vi "Pendel.vi"() -> ()   [LabVIEW 2014]
uses:
  Reglertyp.ctl
  <vilib>/Platform/TimedLoop/XDataNode/timing_clust.ctl
  <vilib>/Platform/TimedLoop/XDataNode/nitl_modes.ctl
  <vilib>/Platform/TimedLoop/XDataNode/wakeup.ctl
  <vilib>/Simulation/Scripting/Companion Diagram/SimConfigNode/SimParams.ctl
  <vilib>/Simulation/Scripting/Companion Diagram/SimConfigNode/_simSolvers.ctl
  <vilib>/Simulation/Implementation/Shared/SIMSCR Execution Mode.ctl
  <vilib>/Simulation/Param Hierarchy/Typedefs/SIMPH Param Control Actions.ctl
  <vilib>/Statechart/Common/IntGuid.ctl
  <vilib>/Statechart/Common/DbgID.ctl
  <vilib>/Analysis/baseanly.llb/Real A x B.vi
  <vilib>/Simulation/Implementation/Shared/NILVSim_ParamChanged.vi
  <vilib>/Simulation/Implementation/Shared/NILVSIM_BeginStep.vi
  <vilib>/Simulation/Implementation/Shared/NILVSim_Manager.vi
  <vilib>/Utility/error.llb/Clear Errors.vi
  <vilib>/Simulation/Implementation/Shared/NILVSim_FinalizeModel.vi
  Pendel.lvsc/CompanionDiagram.vi
  Pendel.lvsc/CompanionDiagram.vi/21/SC Main.vi
  <vilib>/Simulation/Implementation/Shared/SIM Unbundle Sim Info.vi
  <vilib>/Simulation/Implementation/Shared/NILVSim_Initialize.vi
  <vilib>/Simulation/Utility/Implementation/NILVSim Get Time and IsAcceptedStep.vi
  <vilib>/Simulation/Implementation/Shared/SIMSH Read Queue.vi
  <vilib>/Simulation/Implementation/Shared/NILVSim_GetModelError.vi
  <vilib>/Simulation/Implementation/Shared/SIM Bundle Sim Info.vi
  Pendel.lvsc/Trigger.ctl
  <vilib>/Statechart/Infrastructure/RTStatechart/RunTime SCN.xnode
  Pendel.lvsc/Inputs.ctl
  Pendel.lvsc/Outputs.ctl
  Pendel.lvsc
  <vilib>/Platform/TimedLoop/XDataNode/XDataNode.xnode
  <vilib>/Simulation/Implementation/XNodeFramework/SimXNode/SimX.xnode
  <vilib>/Simulation/Scripting/Companion Diagram/SimConfigNode/SimDog.xnode
  <vilib>/Platform/TimedLoop/XDataNode/XDNodeRunTimeDep.lvlib
  <vilib>/Analysis/NI_AALBase.lvlib
  <vilib>/ptbypt/NI_PtbyPt.lvlib
  <vilib>/Statechart/Common/NI_SC_LVSCCommonFiles.lvlib
  <vilib>/Simulation/Implementation/Shared/NI_SIM_Implementation.lvlib
panel:
  out "Winkel 1":dbl
  out "Geschwindigkeit":dbl
  out "Position":dbl
  out "Winkel2":dbl
  out "Winkelgeschwindigkeit2":dbl
  out "Winkelgeschwindigkeit1":dbl
  out "Kraft berechnet":cluster{"Kraft (N)":dbl, dbl}(graph)
  out "Schleifendauer":i64(graph)
  in  "Registerkarte":enum32{"Pendel", "S706", "Wegzähler"}(tab)
  in  "Reglertyp":T1
  in  "Positionieren":bool
  out "Kraft (N)":dbl(graph)
  out "Winkel (Grad)":cluster{"Double":dbl, "Double":dbl}(graph)
  in  "Schließen":bool
  in  "Regler anhalten":bool
  in  "Regler starten":bool
  in  "Ruhelage":bool=TRUE
  in  "Pendelaufbau":T2(ring)
  out "Aktueller Zustand":string
  in  "Referenzieren":bool
  in  "Sollposition (mm)":dbl(slide) scale=-500.0..500.0
  out "Position (mm)":T3(graph)
  out "S706 Status (SDO 6041)":T4
  in  "S706 parametrieren":bool
  out "S706":string
  out "Wegzähler (m)":dbl
  out "Wegzähler (m)":dbl(knob)=6.6072914947233965 scale=5000.0..5000000.0
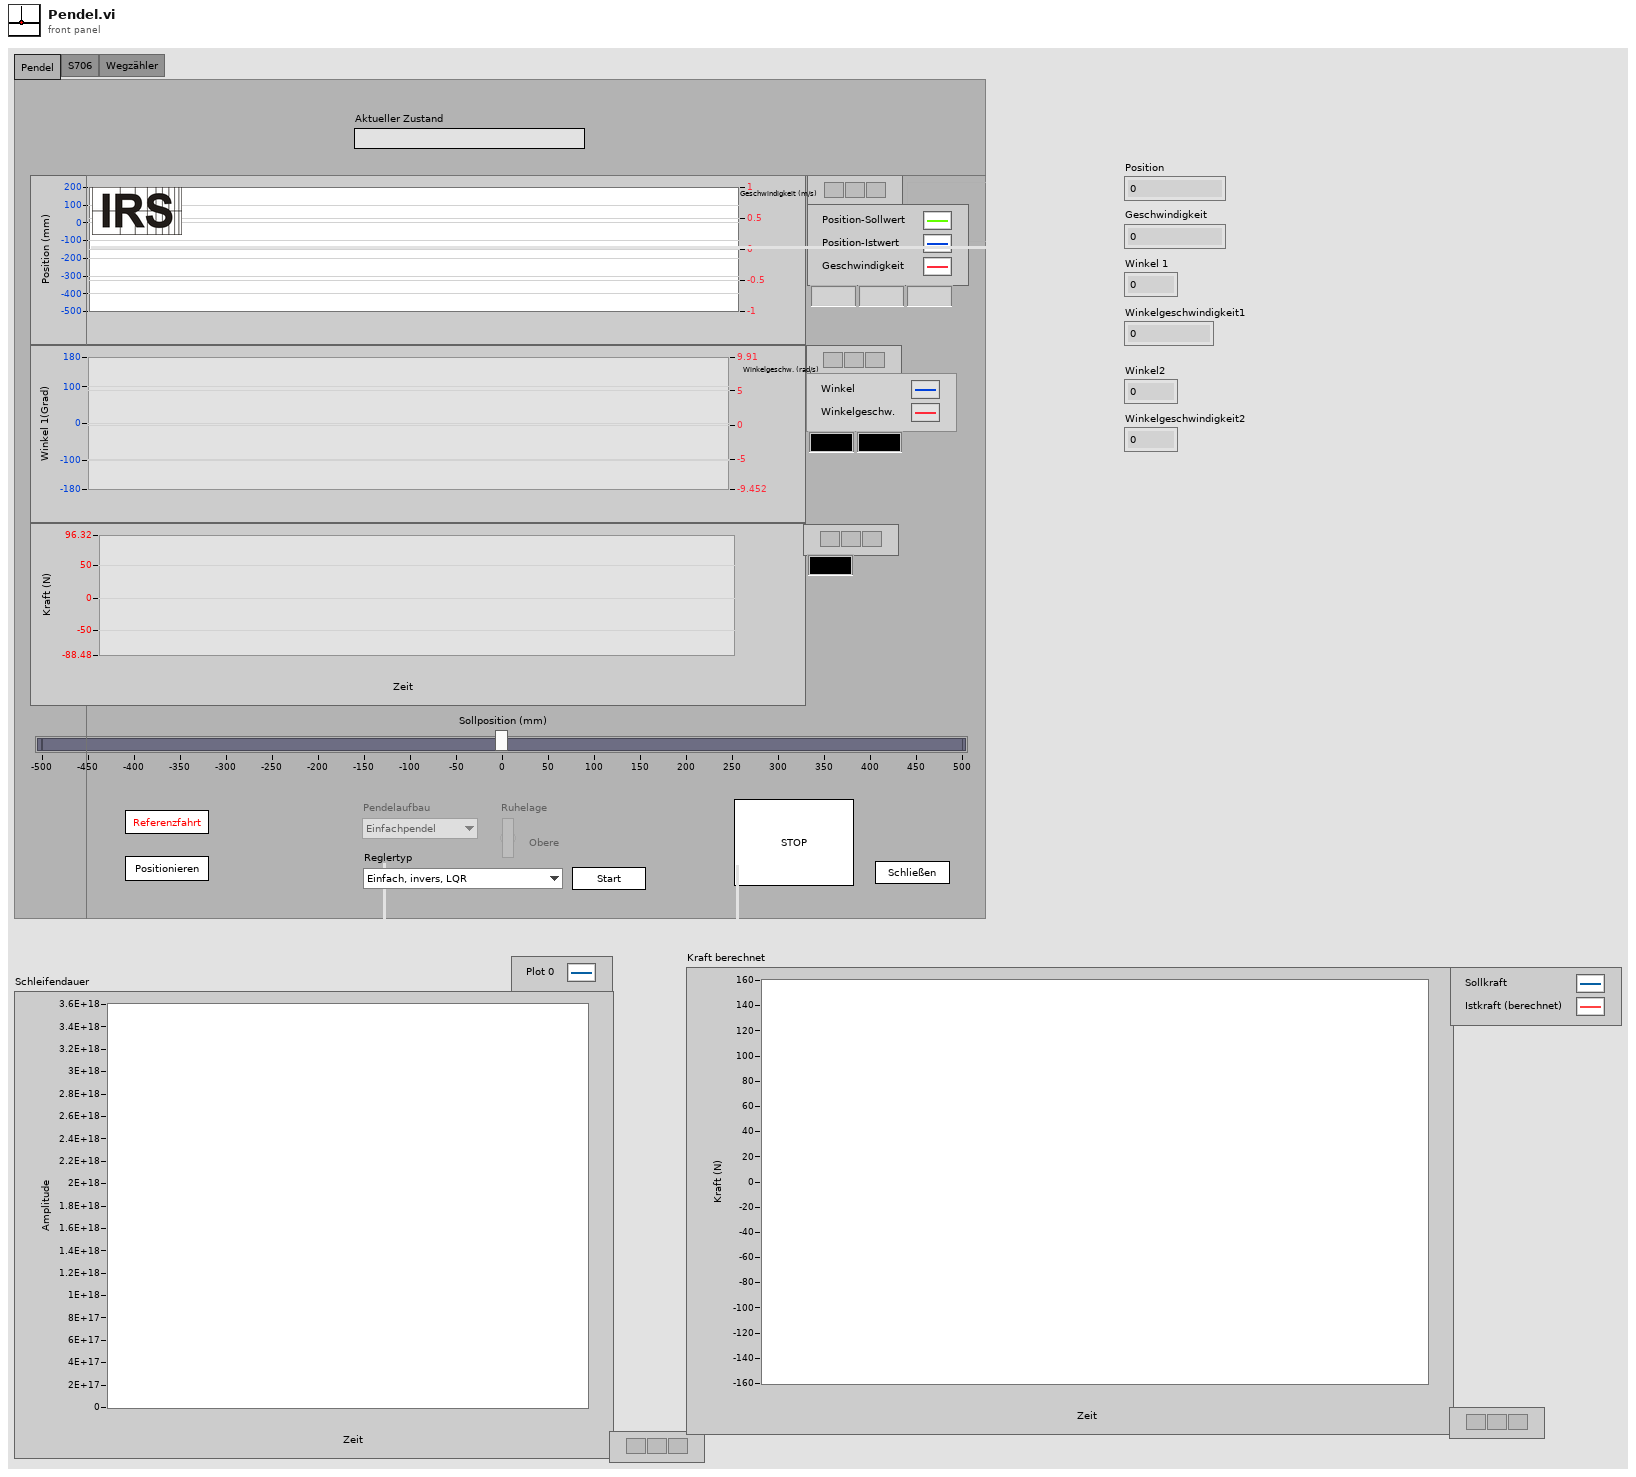
[diagram p1: front panel]
types:
  T1 = typedef "Reglertyp.ctl" = enum16{"Einfach, invers, LQR", "Einfach, invers, Kaskade", "Doppelt, invers, LQR"}
  T2 = enum16{"Einfachpendel", "Doppelpendel", "Dreifachpendel"}
  T3 = cluster{"Sollposition (mm)":dbl, dbl, "Double":dbl}
  T4 = cluster{"0 ready to switch on":bool, "1 switched on":bool, "2 operation enable":bool, "3 fault":bool, "4 voltage enabled":bool, "5 quick stop":bool, "6 switch on disable":bool, "7 warning":bool, "8 ":bool, "9 remote (kann kommunizieren)":bool, "10 target_reached":bool, "11 internal_limit_active":bool, "12 Referenzfahrt durchgeführt":bool, "13 Referenzfahrtfehler":bool}
  T5 = cluster{"Pendelaufbau":enum16{"Einfachpendel", "Doppelpendel", "Dreifachpendel"}, "Winkel1":refnum<k21>, "Winkel2":refnum<k21>, "Winkel3":refnum<k21>}
  T6 = cluster{"node-ID":u8, "RPDO1 controlword":refnum<k20>, "TPDO1 status":refnum<k20>, "RPDO2 I-Sollwert":refnum<k20>, "TPDO2 Ist-Werte":refnum<k20>, "SYNC object":refnum<k20>}
  T7 = typedef "XDNodeRunTimeDep.lvlib/timing_clust.ctl" = cluster{"Expected End [f-1]":u64, "Actual End [f-1]":u64, "Finished Late? [f-1]":bool, "Expected End [i-1]":u64, "Actual End [i-1]":u64, "Finished Late? [i-1]":bool, "Expected Start [i]":u64, "Actual Start [i]":u64, "Expected Start [f]":u64, "Actual Start [f]":u64, "Source Name":string, "Structure Name":string, "Period":i64, "Deadline":i64, "Offset":i64, "Start":i64, "Priority":i32, "Timeout":i32, "Mode":T8, "Wakeup Reason":T9, "Error":errorcluster, "Source Type":string, "Secondary Source Type":string, "Global End Time":u64, "Global Start Time":u64, "Frame Duration":u64, "Iteration Duration":u64, "Assigned CPU":i32, "I/O Scan Engine Mode":u32}
  T8 = typedef "XDNodeRunTimeDep.lvlib/nitl_modes.ctl" = enum32{"No Change", "Process missed periods, maintain original phase", "Discard missed periods, maintain original phase", "Process missed periods, ignore original phase", "Discard missed periods, ignore original phase"}
  T9 = typedef "XDNodeRunTimeDep.lvlib/wakeup.ctl" = enum32{"Normal", "Aborted", "Asynchronous wakeup", "Timing source error", "Timed loop error", "Timeout"}
  T10 = enum16{"Simulate to Completion", "Single Time-Step Simulation (Fixed Step Only)"}
  T11 = typedef "SIMSCR Execution Mode.ctl" = enum16{"Simulate to Completion", "Single Time-Step Simulation (Fixed Step Only)"}
  T12 = typedef "SIMPH Param Control Actions.ctl" = enum16{"get params", "set params"}
  T13 = cluster{"SIMSH Sim Time":dbl, "Saturation":cluster{"output":dbl}, "Derivative":cluster{"output":dbl}, "Integrator":cluster{"output":dbl}, "Transfer Function":cluster{"output y(t)":dbl}, "Summation 7":cluster{"Result":dbl}, "Gain 3":cluster{"output":dbl}, "Gain 2":cluster{"output":dbl}, "Summation 4":cluster{"Result":dbl}, "Summation 6":cluster{"Result":dbl}}
  T14 = typedef "SimParams.ctl" = cluster{"Initial Time (s)":dbl, "Final Time (s)":dbl, "Step Size (s)":dbl, "ODE Solver":T15, "Minimum Step Size (s)":dbl, "Maximum Step Size (s)":dbl, "Relative Tolerance":dbl, "Absolute Tolerance":dbl, "Software Timing":bool, "Initial Step Size (s)":dbl, "Automatic Fixed Step Size?":bool, "Automatic Discrete Step Size?":bool, "Discrete Step Size (s)":dbl, "Calculate using Time Step":bool, "Solver Wired?":bool, "Prev.Frm.Expected End":u64, "Prev.Frm.Actual End":u64, "Prev.Frm.Finished Late?":bool, "Prev.Iter.Expected End":u64, "Prev.Iter.Actual End":u64, "Prev.Iter.Finished Late?":bool, "Expected Iteration Start":u64, "Actual Iteration Start":u64, "Expected Frame Start":u64, "Actual Frame Start":u64, "Source Name":string, "Name":string, "Period":i64, "Deadline":i64, "Offset":i64, "Start":i64, "Priority":i32, "Timeout":i32, "Processor":i32, "Mode":enum32{"No Change", "Process missed periods, maintain original phase", "Discard missed periods, maintain original phase", "Process missed periods, ignore original phase", "Discard missed periods, ignore original phase"}, "Wakeup reason":enum32{"Normal", "Aborted", "Asynchronous wakeup", "Timing source error", "Timed loop error", "Timeout"}, "Error":errorcluster, "Source Type":string, "Secondary Source Type":string, "Global End Time":u64, "Global Start Time":u64, "Full Solver Reset":bool, "Execution Mode":T11, "Nan/Inf Check":bool, "Custom Solver Library":string, "Solver Is Variable":bool, "custom solver name":string, "Signal Collection Decimation":u32}
  T15 = typedef "_simSolvers.ctl" = enum16{"Runge-Kutta 1 (Euler)", "Runge-Kutta 2", "Runge-Kutta 3", "Runge-Kutta 4", "Runge-Kutta 23 (variable)", "Runge-Kutta 45 (variable)", "BDF (variable)", "Adams-Moulton (variable)", "Rosenbrock (variable)", "Discrete States Only", "SDIRK 4 (variable)", "Radau 5 (variable)", "Radau 9 (variable)", "Radau 13 (variable)", "Radau [Variable Order] (variable)", "Gear's Method (variable)", "Linearizer", "State Query", "Trim Eval", "Custom Solver"}
  T16 = cluster{"Winkel1":dbl, "Winkel2":dbl, "Winkel3":dbl}
  T17 = cluster{"Winkelgeschwindigkeit1":dbl, "Winkelgeschwindigkeit2":dbl, "Winkelgeschwindigkeit3":dbl}
  T18 = typedef "NI_Matrix.lvlib/RealMatrix.ctl" = dbl[][]
  T19 = typedef "NI_SC_LVSCCommonFiles.lvlib/IntGuid.ctl" = cluster{"Data1":u32, "Data2":u16, "Data3":u16, "Data4":u8, "Data5":u8, "Data6":u8, "Data11":u8, "Data9":u8, "Data10":u8, "Data8":u8, "Data7":u8}
  T20 = typedef "NI_SC_LVSCCommonFiles.lvlib/DbgID.ctl" = cluster{"VIRef":u32, "IntGUID":T19}
  T21 = enum16{"unbekannt", "Quick stop active", "Fault reaction active", "Fault", "Operation enabled", "Switched on", "Ready to switch on", "Switch on disabled", "Not Ready to switch on"}
  T22 = cluster{bool, bool, bool, bool, bool, bool, bool, bool, bool, bool, bool, bool, bool, bool}
  T23 = cluster{"Positionieren":bool, "Referenzieren":bool, "Regler darf starten":bool, "Regler anhalten":bool, "Schließen":bool, "S706 parametrieren":bool, "error out":errorcluster}
  T24 = typedef "Pendel.lvsc/Outputs.ctl" = cluster{"Zustand":string, "error out":errorcluster}
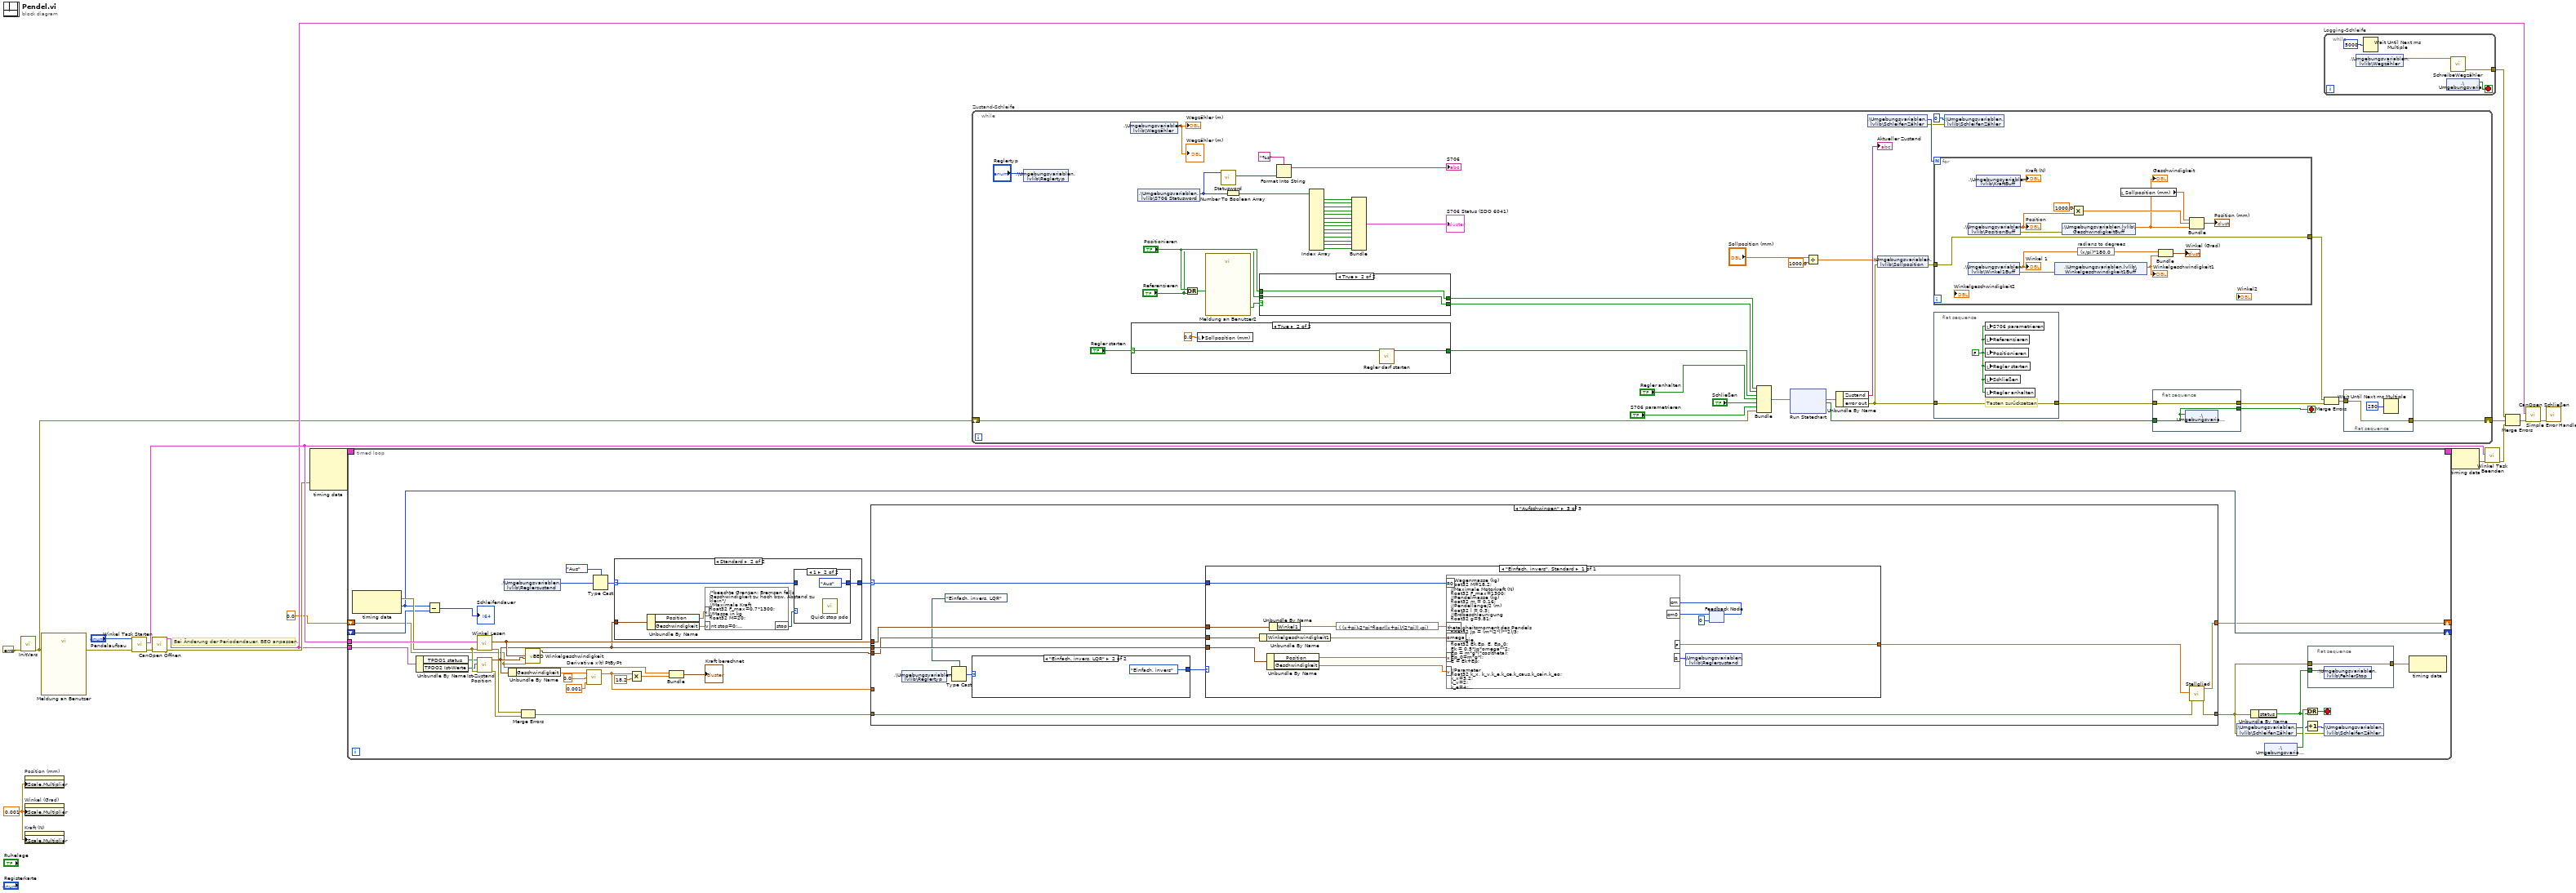
[diagram p0: block diagram]
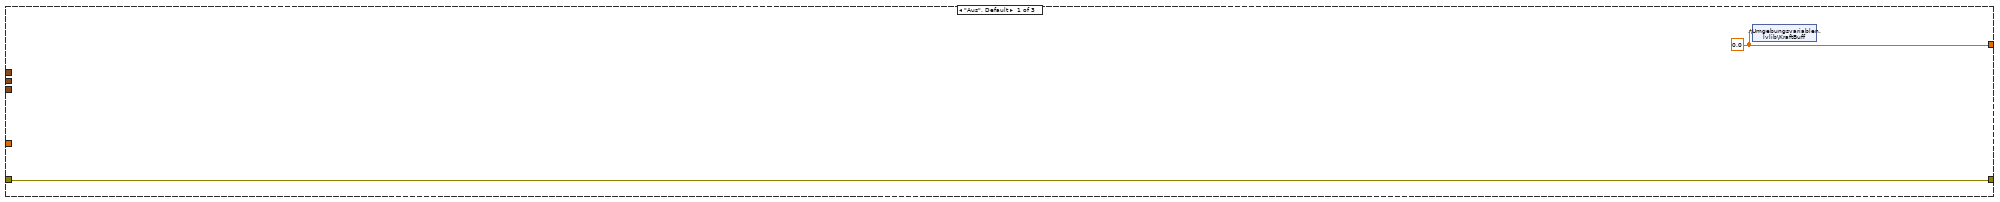
[diagram p4: hidden frame]
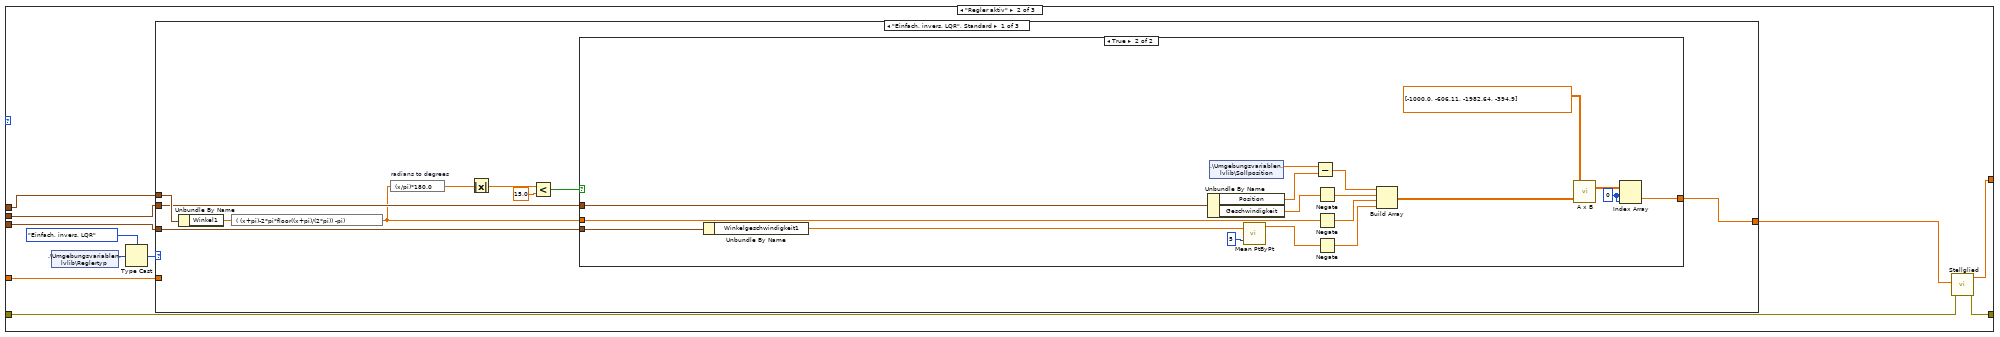
[diagram p5: hidden frame]
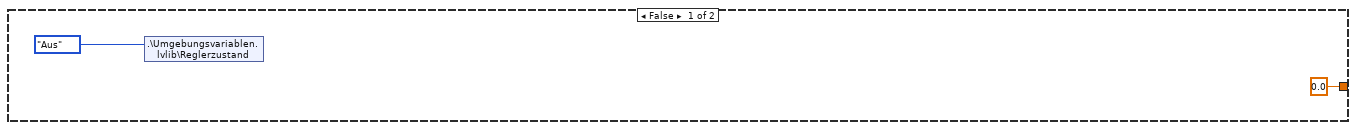
[diagram p6: hidden frame]
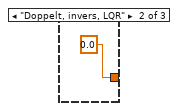
[diagram p7: hidden frame]
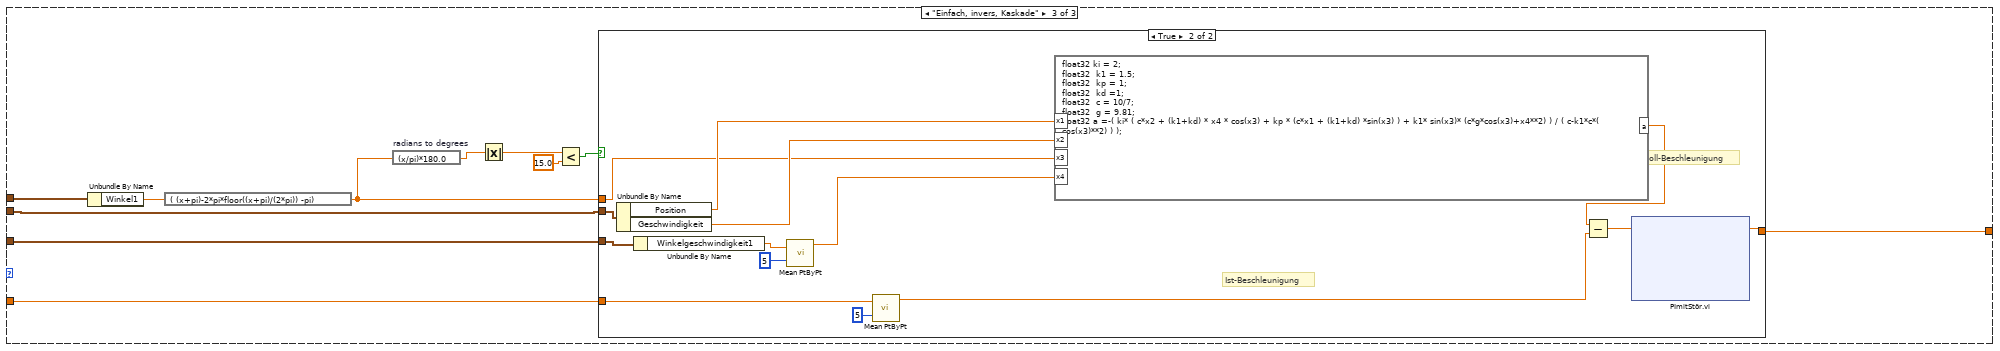
[diagram p8: hidden frame]
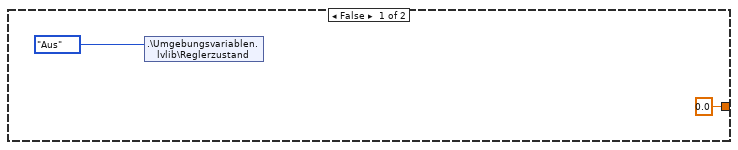
[diagram p9: hidden frame]
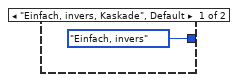
[diagram p10: hidden frame]
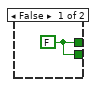
[diagram p11: hidden frame]
diagram:
  w5 = 0.001 ("X-Achse.Offset und Faktor:Faktor")
  # "Bei Änderung der Periodendauer, BEO anpassen."
  n1 = call "InitVars.vi"("error in (no error)"=errorcluster {"status"=FALSE, "code"=0, "source"=""} ("error IO")) -> ("error out"=w4:errorcluster)  [unwired: 10 in]
  n2 = property on="Position (mm)" class="SVDiagr (strikt)"("XScale.Multiplier"=w5) -> ()  [unwired: 2 in, 2 out]
  n3 = property on="Winkel (Grad)" class="SVDiagr (strikt)"("XScale.Multiplier"=w5) -> ()  [unwired: 2 in, 2 out]
  n4 = property on="Kraft (N)" class="SVDiagr (strikt)"("XScale.Multiplier"=w5) -> ()  [unwired: 2 in, 2 out]
  n5 = call "Meldung an Benutzer"("error in (no error)"=w4) -> ("error out"=w10:errorcluster)  [unwired: 9 in, 1 out]
  n6 = call "Winkel Task Starten.vi"("error IO"=w10, "Pendelaufbau in"="Pendelaufbau") -> ("error out"=w2:errorcluster, "Winkel Task"=w13:T5)  [unwired: 8 in]
  n7 = call "CanOpen Öffnen.vi"("error in (no error)"=w2) -> ("Fehler (Ausgang)"=w12:errorcluster, "CanOpen Obj"=w11:T6)  [unwired: 9 in]
  n8 = node-c288(w12) -> (w18:T7)  [unwired: 3 in]
  n9 = timed-loop {
    timing: w18 -> [_]
    timing-out: [_] -> w17
    tunnel: w13 -> [w53]
    tunnel: w11 -> [w48]
    shift-right: [w41] -> _
    shift-left: _ -> [w42]
    shift-right: [w36] -> _
    shift-left: 0.0 ("Kraft (N)") -> [w19]
    stop <- w50 stop-if-true
    n10 = node-c288() -> (w47:errorcluster, w41:i64)  [unwired: 1 in]
    n11 = Unbundle By Name(w48) -> ("TPDO1 status"=w46:refnum<k20>, "TPDO2 Ist-Werte"=w45:refnum<k20>)
    n12 = Subtract(x=w41, y=w42) -> (x-y=→"Schleifendauer":i64)
    n13 = call "Winkel Lesen.vi"("error IO"=w47, "Task In"=w53) -> ("error out"=w43:errorcluster, "Winkel"=w21:T16)  [unwired: 8 in]
    n14 = call "Ist-Zustand Position.vi"("Fehler (Eingang, kein Fehler)"=w47, "TPDO2 object in"=w45, "TPDO1 object in"=w46) -> ("error out"=w44:errorcluster, "Ist-Zustand Position"=w20:cluster{"Position":dbl, "Geschwindigkeit":dbl})  [unwired: 7 in]
    n15 = shared-variable ".\\Umgebungsvariablen.lvlib\\Reglerzustand"() -> (w30:u16)  [unwired: 1 in, 1 out]
    n16 = Unbundle By Name(w20) -> ("Geschwindigkeit"=w32:dbl)
    n17 = Merge Errors(w43, w44) -> (w51:errorcluster)
    n18 = call "BEO Winkelgeschwindigkeit.vi"("Kraft (N)"=w19, "Ist-Zustand Position (m, m/s)"=w20, "Winkel (rad)"=w21) -> ("Winkelgeschwindigkeit (1/s)"=w22:T17)  [unwired: 8 in]
    n19 = call <vilib>:"Derivative x(t) PtByPt.vi"("dt"=0.001, "initial condition"=0.0, "x"=w32) -> ("dx/dt"=w23:dbl)  [unwired: 1 in, 1 out]
    n20 = Type Cast(type=enum16{"Aus", "Aufschwingen", "Regler aktiv"}."Aus", x=w30) -> (*(type *) &x=w26:enum16{"Aus", "Aufschwingen", "Regler aktiv"})
    n21 = case shown="Standard" w26 {
      selector: w26 -> [w54 w56]
      tunnel: [w54 w55] -> w25
      tunnel: w20 -> [_ w60]
      frame "Aus" {
      }
      frame Default {
        n22 = Unbundle By Name(w60) -> ("Position"=w58:dbl, "Geschwindigkeit"=w59:dbl)
        n23 = formula code="/*beachte Grenzen: Bremsen falls Geschwindigkeit zu hoch bzw. Abstand zu klein*/\n//Maximale Kraft\nfloat32 F_max=0.7*1300;\n//Masse in kg\nfloat32 M=20;\n\nint stop=0;\nif((abs(x)+0.5*M/F_max*v**2)>=0.75)\nstop=1;"("x"=w58, "v"=w59) -> ("stop"=w57:i32)
        n24 = case shown="1" w57 {
          tunnel: w56 -> [w61 _]
          tunnel: [w61 enum16{"Aus", "Aufschwingen", "Regler aktiv"}."Aus"] -> w55
          frame 0, Default {
          }
          frame 1 {
            n25 = call "Quick stop pdo.vi"() -> ()  [unwired: 11 in, 1 out]
          }
        }
      }
    }
    n26 = Multiply(x=w23, y=18.2) -> (x*y=w24:dbl)
    n27 = Bundle("Kraft (N)"=w19, w24) -> (→"Kraft berechnet":cluster{"Kraft (N)":dbl, dbl})  [unwired: 1 in]
    n28 = case shown="\"Aufschwingen\"" w25 {
      selector: w25 -> [_ _ w383]
      tunnel: w21 -> [_ w77 w384]
      tunnel: w20 -> [_ w73 w385]
      tunnel: w22 -> [_ w76 w382]
      tunnel: w51 -> [w66 w71 w386]
      tunnel: [w66 w75 w388] -> w28
      tunnel: [w65 w72 w387] -> w36
      tunnel: w23 -> [_ w67 _]
      frame "Aus", Default {
        w65 = 0.0 ("Kraft (N)")
        n29 = shared-variable ".\\Umgebungsvariablen.lvlib\\KraftBuff"(w65) -> ()  [unwired: 1 in, 1 out]
      }
      frame "Regler aktiv" {
        n30 = shared-variable ".\\Umgebungsvariablen.lvlib\\Reglertyp"() -> (w70:i16)  [unwired: 1 in, 1 out]
        n31 = Type Cast(type=Reglertyp."Einfach, invers, LQR" ("Regler"), x=w70) -> (*(type *) &x=w68:T1)
        n32 = case shown="\"Einfach, invers, LQR\", Standard" w68 {
          tunnel: w77 -> [w87 _ w119]
          tunnel: [w84 0.0 ("Real Matrix Element") w109] -> w74
          tunnel: w76 -> [w86 _ w113]
          tunnel: w73 -> [w85 _ w111]
          tunnel: w67 -> [_ _ w110]
          frame "Einfach, invers, LQR", Default {
            n33 = Unbundle By Name(w87) -> ("Winkel1"=w79:dbl)
            n34 = expression code="( (x+pi)-2*pi*floor((x+pi)/(2*pi)) -pi)" ("Ausdrucksknoten")(w79) -> (w78:dbl)
            n35 = expression code="(x/pi)*180.0" "radians to degrees"(w78) -> (w81:dbl)
            n36 = Absolute Value(x=w81) -> (abs(x)=w82:dbl)
            n37 = Less?(x=w82, y=15.0) -> (x < y?=w83:bool)
            n38 = case shown="True" w83 {
              tunnel: w86 -> [_ w107]
              tunnel: w85 -> [_ w106]
              tunnel: w78 -> [_ w105]
              tunnel: [0.0 ("Real Matrix Element") w98] -> w84
              frame False {
                n39 = shared-variable ".\\Umgebungsvariablen.lvlib\\Reglerzustand"(enum16{"Aus", "Aufschwingen", "Regler aktiv"}."Aus") -> ()  [unwired: 1 in, 1 out]
              }
              frame True {
                w100 = 0 ("Index (Zeile)")
                n40 = Unbundle By Name(w107) -> ("Winkelgeschwindigkeit1"=w94:dbl)
                n41 = Unbundle By Name(w106) -> ("Position"=w102:dbl, "Geschwindigkeit"=w104:dbl)
                n42 = shared-variable ".\\Umgebungsvariablen.lvlib\\Sollposition"() -> (w103:dbl)  [unwired: 1 in, 1 out]
                n43 = call <vilib>:"Mean PtByPt.vi"("x"=w94, "sample length"=5) -> ("mean"=w93:dbl)  [unwired: 2 in, 1 out]
                n44 = Subtract(x=w103, y=w102) -> (x-y=w95:dbl)
                n45 = Negate(x=w104) -> (-x=w91:dbl)
                n46 = Negate(x=w105) -> (-x=w96:dbl)
                n47 = Negate(x=w93) -> (-x=w97:dbl)
                n48 = Build Array(w95, w91, w96, w97) -> (w101:T18)
                n49 = call-poly <vilib>:"A x B.vi"("B"=w101, "A"=dbl[][] [[-1000.0, -606.11, -1982.64, -394.9]]) -> ("A x B"=w99:T18)  [unwired: 1 out]
                n50 = Index Array(array=w99, index (row)=w100, index (col)=w100) -> (element=w98:dbl)
              }
            }
          }
          frame "Doppelt, invers, LQR" {
          }
          frame "Einfach, invers, Kaskade" {
            n51 = Unbundle By Name(w119) -> ("Winkel1"=w118:dbl)
            n52 = expression code="( (x+pi)-2*pi*floor((x+pi)/(2*pi)) -pi)" ("Ausdrucksknoten")(w118) -> (w112:dbl)
            n53 = expression code="(x/pi)*180.0" "radians to degrees"(w112) -> (w115:dbl)
            n54 = Absolute Value(x=w115) -> (abs(x)=w117:dbl)
            n55 = Less?(x=w117, y=15.0) -> (x < y?=w114:bool)
            n56 = case shown="True" w114 {
              tunnel: w113 -> [_ w135]
              tunnel: w112 -> [_ w130]
              tunnel: w111 -> [_ w134]
              tunnel: w110 -> [_ w125]
              tunnel: [0.0 ("F") w122] -> w109
              frame False {
                n57 = shared-variable ".\\Umgebungsvariablen.lvlib\\Reglerzustand"(enum16{"Aus", "Aufschwingen", "Regler aktiv"}."Aus") -> ()  [unwired: 1 in, 1 out]
              }
              frame True {
                # "Soll-Beschleunigung"
                # "Ist-Beschleunigung"
                n58 = Unbundle By Name(w134) -> ("Position"=w133:dbl, "Geschwindigkeit"=w131:dbl)
                n59 = Unbundle By Name(w135) -> ("Winkelgeschwindigkeit1"=w127:dbl)
                n60 = call <vilib>:"Mean PtByPt.vi"("x"=w127, "sample length"=5) -> ("mean"=w128:dbl)  [unwired: 2 in, 1 out]
                n61 = call <vilib>:"Mean PtByPt.vi"("x"=w125, "sample length"=5) -> ("mean"=w124:dbl)  [unwired: 2 in, 1 out]
                n62 = formula code="float32 ki = 2;\nfloat32  k1 = 1.5;\nfloat32  kp = 1;\nfloat32  kd =1;\nfloat32  c = 10/7;\nfloat32  g = 9.81;\nfloat32 a =-( ki* ( c*x2 + (k1+kd) * x4 * cos(x3) + kp * (c*x1 + (k1+kd) *sin(x3) ) + k1* sin(x3)* (c*g*cos(x3)+x4**2) ) / ( c-k1*c*( cos(x3)**2) ) );" ("Formelknoten")("x1"=w133, "x2"=w131, "x3"=w130, "x4"=w128) -> ("a"=w132:sgl)
                n63 = Subtract(x=w132, y=w124) -> (x-y=w123:dbl)
                n64 = xnode "PImitStör.vi"("a"=w123) -> ("F"=w122:dbl)  [unwired: 2 in, 11 out]
              }
            }
          }
        }
        n65 = call "Stellglied.vi"("error in (no error)"=w71, "Stellgröße - Kraft (N)"=w74) -> ("error out"=w75:errorcluster, "Kraft (N)"=w72:dbl)  [unwired: 8 in]
      }
      frame "Aufschwingen" {
        n66 = shared-variable ".\\Umgebungsvariablen.lvlib\\Reglertyp"() -> (w380:i16)  [unwired: 1 in, 1 out]
        n67 = Type Cast(type=Reglertyp."Einfach, invers, LQR" ("Regler"), x=w380) -> (*(type *) &x=w379:T1)
        n68 = case shown="\"Einfach, invers, LQR\"" w379 {
          tunnel: [enum16{"Einfach, invers"}."Einfach, invers" enum16{"Einfach, invers"}."Einfach, invers"] -> w378
          frame "Einfach, invers, Kaskade", Default {
          }
          frame "Einfach, invers, LQR" {
          }
        }
        n69 = case shown="\"Einfach, invers\", Standard" w378 {
          tunnel: w385 -> [w395]
          tunnel: w384 -> [w394]
          tunnel: w383 -> [w393]
          tunnel: w382 -> [w392]
          tunnel: [w391] -> w381
          frame "Einfach, invers", Default {
            n70 = Unbundle By Name(w392) -> ("Winkelgeschwindigkeit1"=w403:dbl)
            n71 = Unbundle By Name(w395) -> ("Position"=w402:dbl, "Geschwindigkeit"=w404:dbl)
            n72 = Unbundle By Name(w394) -> ("Winkel1"=w400:dbl)
            n73 = expression code="( (x+pi)-2*pi*floor((x+pi)/(2*pi)) -pi)" ("Ausdrucksknoten")(w400) -> (w401:dbl)
            n74 = feedback #1 ("Rückkopplungsknoten")(0) -> (w397:i32)
            n75 = formula code="//Wagenmasse (kg)\nfloat32 M=18.2;\n//Maximale Motorkraft (N)\nfloat32 F_max=1300;\n//Pendelmasse (kg)\nfloat32 m = 0.16; \n//Pendellänge/2 (m)\nfloat32 l = 0.3; \n//Erdbeschleunigung\nfloat32 g=9.81;\n\n//Trägheitsmoment des Pendels\nfloat32 Jp = (m*(2*l)**2)/3;\n\n//Energie\nfloat32 Ek,Ep, E, Ep_0;\nEk = 0.5*Jp*omega**2;\nEp = m*g*l*cos(theta);\nEp_0=m*g*l;\nE = Ek+Ep;\n\n//Parameter\nfloat32 k_x, k_v,k_e,k_ce,k_caus,k_cein,k_eo;\nk_x=3.2;\nk_v=2;\nk_e=4;\nk_ce=4;\nk_caus=0.75;\nk_cein=1;\nk_eo=1;\n//k_eo=1.05;\n\n//Potentialtopf - Position\nfloat32 u_x;\nif(abs(x)<0.6)\nu_x=k_x*sign(x)*ln(1-abs(x)/0.6);\nelse\nu_x=-F_max/M*sign(x);\n\n//Potentialtopf - Geschwindigkeit\nfloat32 u_v;\nif(abs(v)<6)\nu_v=k_v*sign(v)*ln(1-abs(v)/6);\nelse\nu_v=-F_max/M*sign(v);\n\nint cm;\nif(E>k_cein*Ep_0) \ncm=1;\nelse if (E<k_caus*Ep_0) \ncm=0;\nelse\ncm=cm0;\n\nfloat32 u, F;\nif(cm)\nu=u_x + u_v+k_ce*(E-k_eo*Ep_0)*sign(omega*cos(theta));\n//u=u_x + u_v+k_ce*(exp(abs(E-k_eo*Ep_0))-1)*sign(E-Ep_0)*sign(omega*cos(theta));\nelse\nu=-k_e*sign(omega*cos(theta))+u_x;\nu=2*u;\nF=(Jp*(M+m)-(m*l)**2*cos(theta)**2)/Jp*u-m*l*sin(theta)*omega**2+(m*l)**2*g*sin(theta)*cos(theta)/Jp;\n\n/*Regler aktivieren?*/\nint R=1; //Regelzustand: Aufschwingen\nif( abs(theta)/pi*180<10 && abs(x)<0.4 && abs(omega)<1 || (R0==1 &&abs(theta)/pi*180<15))\nR=2; //Reglerzustand: Regler aktiviert"("x"=w402, "v"=w404, "theta"=w401, "omega"=w403, "cm0"=w397, "R0"=w393) -> ("F"=w391:sgl, "cm"=w396:i32, "R"=w399:i32)
            n76 = shared-variable ".\\Umgebungsvariablen.lvlib\\Reglerzustand"(w399) -> ()  [unwired: 1 in, 1 out]
            n77 = feedback-in #1 ("2")(w396) -> ()
          }
        }
        n78 = call "Stellglied.vi"("error in (no error)"=w386, "Stellgröße - Kraft (N)"=w381) -> ("error out"=w388:errorcluster, "Kraft (N)"=w387:dbl)  [unwired: 8 in]
      }
    }
    n79 = shared-variable ".\\Umgebungsvariablen.lvlib\\SchleifenZähler"(error in=w28) -> (w34:u16, error out=w33:errorcluster)
    n80 = Unbundle By Name(w28) -> ("status"=w29:bool)
    n81 = shared-variable ".\\Umgebungsvariablen.lvlib\\stop"() -> (w49:bool)  [unwired: 1 in, 1 out]
    n82 = Or(x=w49, y=w29) -> (x .or. y?=w50:bool)
    n83 = Increment(x=w34) -> (x+1=w35:u16)
    n84 = flat-sequence {
      tunnel: w29 -> [w64]
      tunnel: w28 -> [w63]
      tunnel: [w63] -> w27
      frame #0 {
        n85 = shared-variable ".\\Umgebungsvariablen.lvlib\\FehlerStop"(w64) -> ()  [unwired: 1 in, 1 out]
      }
    }
    n86 = shared-variable ".\\Umgebungsvariablen.lvlib\\SchleifenZähler"(w35, error in=w33) -> ()  [unwired: 1 out]
    n87 = node-c288(w27) -> ()  [unwired: 1 out]
  }
  n88 = while "Zustand-Schleife" {
    shift-right: [w454] -> w16
    shift-left: w4 -> [w435]
    stop <- w456 stop-if-true
    n89 = shared-variable ".\\Umgebungsvariablen.lvlib\\Reglertyp"("Reglertyp") -> ()  [unwired: 1 in, 1 out]
    n90 = shared-variable ".\\Umgebungsvariablen.lvlib\\Wegzähler"() -> (→"Wegzähler (m)" →"Wegzähler (m)":dbl)  [unwired: 1 in, 1 out]
    n91 = case shown="True" "Regler starten" {
      selector: "Regler starten" -> [w466 w468]
      tunnel: [w466 w467] -> w419
      frame False {
      }
      frame True {
        n92 = local write "Sollposition (mm)"(0.0 ("Sollposition (mm)")) -> ()
        n93 = call "Regler darf starten.vi"("Regler start"=w468) -> ("Regler darf starten"=w467:bool)  [unwired: 10 in]
      }
    }
    n94 = shared-variable ".\\Umgebungsvariablen.lvlib\\S706 Statusword"() -> (w451:u16)  [unwired: 1 in, 1 out]
    n95 = Or(x="Positionieren", y="Referenzieren") -> (x .or. y?=w418:bool)
    n96 = call "Meldung an Benutzer2"("Enable"=w418) -> ("OK"=w417:bool)  [unwired: 9 in, 1 out]
    n97 = call "Statusword.vi"("Wert"=w451) -> ("Status"=w426:T21)  [unwired: 10 in]
    n98 = Number To Boolean Array(number=w451) -> (Boolean array=w452:bool[])
    n99 = case shown="True" w417 {
      tunnel: "Referenzieren" -> [_ w464]
      tunnel: "Positionieren" -> [_ w465]
      tunnel: [w463 w465] -> w415
      tunnel: [w463 w464] -> w413
      frame False {
        w463 = FALSE ("Positionieren")
      }
      frame True {
      }
    }
    n100 = Format Into String(format string="%s" ("Format-String"), w426) -> (resulting string=→"S706":string)  [unwired: 2 in, 1 out]
    n101 = Index Array(array=w452) -> (element #1=w450:bool, element #2=w449:bool, element #3=w448:bool, element #4=w447:bool, element #5=w446:bool, element #6=w445:bool, element #7=w444:bool, element #8=w443:bool, element #9=w442:bool, element #10=w441:bool, element #11=w440:bool, element #12=w439:bool, element #13=w438:bool, element #14=w437:bool)  [unwired: 14 in]
    n102 = Bundle(w450, w449, w448, w447, w446, w445, w444, w443, w442, w441, w440, w439, w438, w437) -> (→"S706 Status (SDO 6041)":T22)  [unwired: 1 in]
    n103 = Bundle("Positionieren"=w415, "Referenzieren"=w413, "Regler darf starten"=w419, "Regler anhalten"="Regler anhalten", "Schließen"="Schließen", "S706 parametrieren"="S706 parametrieren", "error out"=w435) -> (w457:T23)  [unwired: 1 in]
    n104 = xnode "Run Statechart"("Inputs"=w457) -> ("Terminated?"=w458:bool, "Outputs"=w460:T24)  [unwired: 2 in]
    n105 = Divide(x="Sollposition (mm)", y=1000.0) -> (x/y=w429:dbl)
    n106 = Unbundle By Name(w460) -> ("Zustand"=→"Aktueller Zustand":string, "error out"=w420:errorcluster)
    n107 = shared-variable ".\\Umgebungsvariablen.lvlib\\SchleifenZähler"() -> (w432:u16, error out=w430:errorcluster)  [unwired: 1 in]
    n108 = shared-variable ".\\Umgebungsvariablen.lvlib\\Sollposition"(w429, error in=w420) -> (error out=w421:errorcluster)
    n109 = for {
      N: w432 -> [_]
      tunnel: w421 -> [w475]
      tunnel: [w475] -> w434
      n110 = shared-variable ".\\Umgebungsvariablen.lvlib\\PositionBuff"() -> (w480:dbl, error out=w474:errorcluster)  [unwired: 1 in]
      "Position" <- w480
      n111 = shared-variable ".\\Umgebungsvariablen.lvlib\\Winkel1Buff"() -> (w477:dbl, error out=w478:errorcluster)  [unwired: 1 in]
      "Winkel 1" <- w477
      n112 = shared-variable ".\\Umgebungsvariablen.lvlib\\KraftBuff"() -> (→"Kraft (N)":dbl)  [unwired: 1 in, 1 out]
      n113 = shared-variable ".\\Umgebungsvariablen.lvlib\\Winkelgeschwindigkeit1Buff"(error in=w478) -> (w470:dbl)  [unwired: 1 out]
      "Winkelgeschwindigkeit1" <- w470
      n114 = shared-variable ".\\Umgebungsvariablen.lvlib\\GeschwindigkeitBuff"(error in=w474) -> (w472:dbl)  [unwired: 1 out]
      "Geschwindigkeit" <- w472
      n115 = Multiply(x=1000.0, y=w480) -> (x*y=w482:dbl)
      n116 = expression code="(x/pi)*180.0" "radians to degrees"(w477) -> (w473:dbl)
      n117 = local read "Sollposition (mm)"() -> (w471:dbl)
      n118 = Bundle("Double"=w473, "Double"=w470) -> (→"Winkel (Grad)":cluster{"Double":dbl, "Double":dbl})  [unwired: 1 in]
      n119 = Bundle("Sollposition (mm)"=w471, w482, "Double"=w472) -> (→"Position (mm)":T3)  [unwired: 1 in]
    }
    n120 = flat-sequence {
      tunnel: [w489] -> w433
      tunnel: w420 -> [w489]
      frame #0 {
        w488 = FALSE
        # "Tasten zurücksetzen"
        n121 = local write "S706 parametrieren"(w488) -> ()
        n122 = local write "Referenzieren"(w488) -> ()
        n123 = local write "Positionieren"(w488) -> ()
        n124 = local write "Regler starten"(w488) -> ()
        n125 = local write "Schließen"(w488) -> ()
        n126 = local write "Regler anhalten"(w488) -> ()
      }
    }
    n127 = shared-variable ".\\Umgebungsvariablen.lvlib\\SchleifenZähler"(u16 0 ("SchleifenZähler"), error in=w430) -> ()  [unwired: 1 out]
    n128 = flat-sequence {
      tunnel: w433 -> [w486]
      tunnel: [w486] -> w423
      tunnel: w458 -> [w487]
      tunnel: [w487] -> w456
      frame #0 {
        n129 = shared-variable ".\\Umgebungsvariablen.lvlib\\stop"(w487) -> ()  [unwired: 1 in, 1 out]
      }
    }
    n130 = Merge Errors(w434, w423) -> (w455:errorcluster)
    n131 = flat-sequence {
      tunnel: [w485] -> w454
      tunnel: w455 -> [w485]
      frame #0 {
        n132 = Wait Until Next ms Multiple(millisecond multiple=u32 250 ("ms")) -> ()  [unwired: 1 out]
      }
    }
  }
  n133 = while "Logging-Schleife" {
    tunnel: [w509] -> w1
    stop <- w507 stop-if-true
    n134 = shared-variable ".\\Umgebungsvariablen.lvlib\\Wegzähler"() -> (w510:dbl)  [unwired: 1 in, 1 out]
    n135 = Wait Until Next ms Multiple(millisecond multiple=u32 5000 ("ms")) -> ()  [unwired: 1 out]
    n136 = shared-variable ".\\Umgebungsvariablen.lvlib\\stop"() -> (w507:bool)  [unwired: 1 in, 1 out]
    n137 = call "SchreibeWegzähler.vi"("Aktuell"=w510) -> ("error out"=w509:errorcluster)  [unwired: 10 in]
  }
  n138 = node-c288(w17) -> (w15:errorcluster)
  n139 = call "Winkel Task Beenden.vi"("error IO"=w15, "Task In"=w13) -> ("error out"=w8:errorcluster)  [unwired: 9 in]
  n140 = Merge Errors(w1, w16, w8) -> (w7:errorcluster)
  n141 = call "CanOpen Schließen.vi"("error in (no error)"=w7, "CanOpen Obj"=w11) -> ("Fehler (Ausgang)"=w6:errorcluster)  [unwired: 9 in]
  n142 = call <vilib>:"Simple Error Handler.vi"("error in (no error)"=w6) -> ()  [unwired: 4 in, 5 out]
